vi "PAQ_getPointers.vi"(7 "Layer":i32, 8 "error in (no error)":errorcluster, 11 "FAMM in":refnum<class "FAMM.lvclass">) -> (0 "error out":errorcluster, 1 "Pointers":cluster{"Pointer":i32, "Carry":i32}, 3 "FAMM out":refnum<class "FAMM.lvclass">)   [LabVIEW 2020, in "FAMM.lvclass"]
doc: "Get PAQ memory layer pointers"
uses:
  FAMM.lvclass
  PAQ-memory.lvclass
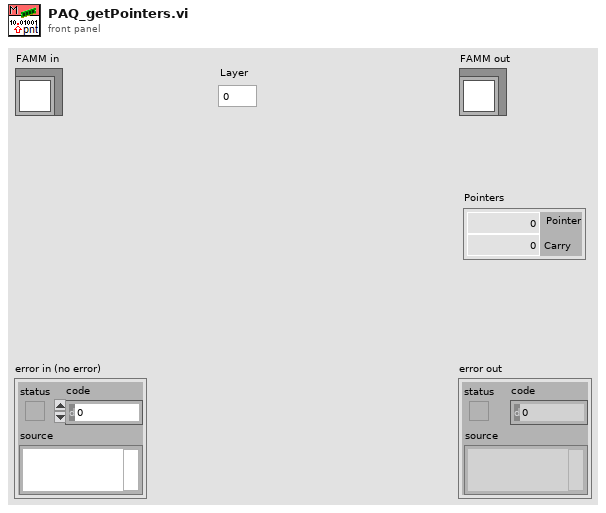
[diagram p1: front panel]
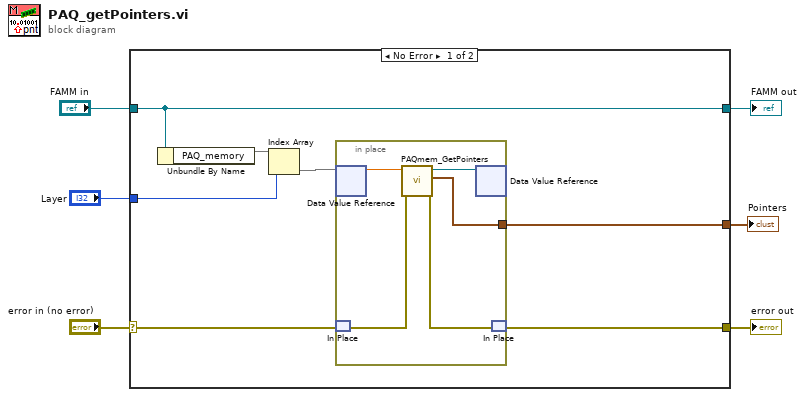
[diagram p0: block diagram]
diagram:
  n1 = case shown="No Error" "error in (no error)" {
    selector: "error in (no error)" -> [w8 w20]
    tunnel: [w7 w20] -> w5
    tunnel: [w13 w19] -> w3
    tunnel: "FAMM in" -> [w13 w19]
    tunnel: "Layer" -> [w11 _]
    tunnel: [w9 _] -> w1
    frame No Error {
      n2 = Unbundle By Name(w13) -> ("PAQ_memory"=w12)
      n3 = Index Array(array=w12, index=w11) -> (element=w10)
      n4 = in-place {
        in-place-border: [w16] -> w9
        n5 = in-place-dvr #1(w10) -> (w18:dbl)  [unwired: 1 out]
        n6 = in-place-match #2(w8) -> (w15:errorcluster)
        n7 = call "PAQmem_GetPointers.vi"("error in (no error)"=w15, "PAQ-memory in"=w18) -> ("error out"=w14:errorcluster, "Pointers"=w16:cluster{"Pointer":i32, "Carry":i32}, "PAQ-memory out"=w17:refnum<class "PAQ-memory.lvclass">)  [unwired: 7 in]
        n8 = in-place-dvr #1(w17) -> ()  [unwired: 2 out]
        n9 = in-place-match #2(w14) -> (w7:errorcluster)
      }
    }
    frame Error {
    }
  }
  "error out" <- w5
  "FAMM out" <- w3
  "Pointers" <- w1
